vi "Close.vi"(8 "error in (no error)":errorcluster, 11 "Data in":refnum<class "Event_Bus.lvclass">) -> (0 "error out":errorcluster, 3 "Data out":refnum<class "Event_Bus.lvclass">)   [LabVIEW 2021, in "Event_Bus.lvclass"]
doc: "Abstract Data Classes 2.1.1.13\nTim Streeter - TSA\nCopyright (c) 2025, TSA"
uses:
  Event_Bus.lvclass
  Event_Bus.lvclass/Event_Bus.ctl
  Properties/Read Event_Source.vi
  Properties/Read Buses.vi
  Support/Event Source/Event_Source.lvclass
  Omni-Bus/Bus Access/Bus_Access.lvclass
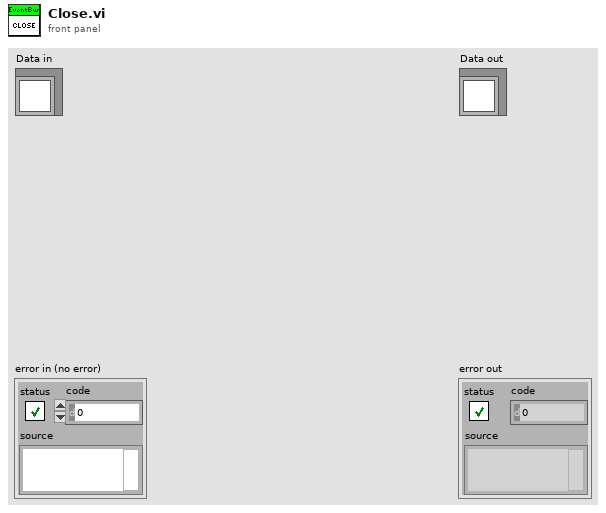
[diagram p1: front panel]
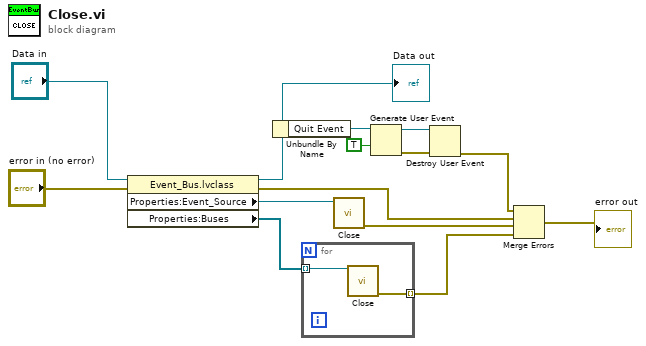
[diagram p0: block diagram]
diagram:
  n1 = property class="Event_Bus.lvclass"(reference="Data in", error in="error in (no error)") -> (reference out=w7:refnum<class "Event_Bus.lvclass">, error out=w5:errorcluster, "Properties:Event_Source"=w12:refnum<class "Event_Source.lvclass">, "Properties:Buses"=w11:refnum<class "Bus_Access.lvclass">[])
  "Data out" <- w7
  n2 = Unbundle By Name(w7) -> ("Quit Event"=w6:refnum<user-event>)
  n3 = for {
    tunnel: w11 -> [w16] mode=indexing
    tunnel: [w15] -> w9 mode=indexing
    n4 = call-dynamic "Close.vi"("Data in"=w16) -> ("error out"=w15:errorcluster)  [unwired: 9 in, 1 out]
  }
  n5 = call-dynamic "Close.vi"("Data in"=w12) -> ("error out"=w10:errorcluster)  [unwired: 9 in, 1 out]
  n6 = Generate User Event(user event=w6, event data cluster=TRUE ("event data")) -> (user event out=w3:refnum<user-event>, error out=w1:errorcluster)  [unwired: 2 in]
  n7 = Destroy User Event(user event=w3, error in=w1) -> (error out=w2:errorcluster)
  n8 = Merge Errors(w2, w5, w10, w9) -> (→"error out":errorcluster)
